vi "Generate Process.vi"(8 "error in (no error)":errorcluster, 11 "Process Generator In":refnum<class "Process Generator.lvclass">) -> (0 "error out":errorcluster, 3 "Process Generator Out":refnum<class "Process Generator.lvclass">)   [LabVIEW 2020, in "Process Generator.lvclass"]
uses:
  Process Generator.lvclass
  Process Generator.lvclass/Process Generator.ctl
  Framework/Process/Process.lvclass
  C:/Users/anton/Documents/GitHub/Triarc-Framework/source/Framework/Base/Base.lvclass
  C:/Users/anton/Documents/GitHub/Triarc-Framework/source/Framework/Configuration File/Configuration File.lvclass
  C:/Users/anton/Documents/GitHub/Triarc-Framework/source/Framework/Process/Process.lvclass
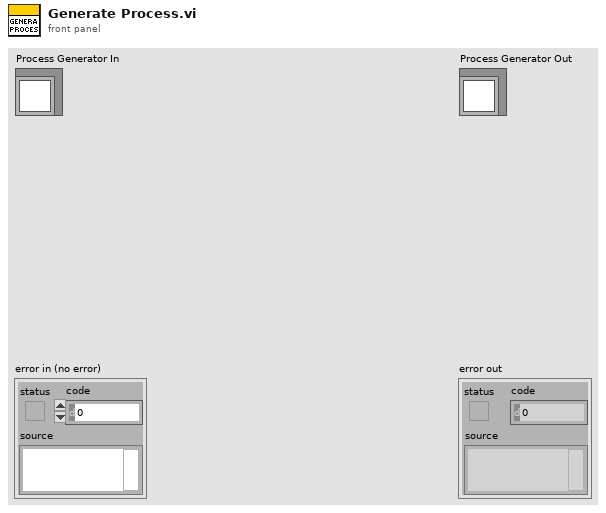
[diagram p1: front panel]
types:
  T1 = enum32{"invalid scope", "public", "private", "protected", "community"}[]
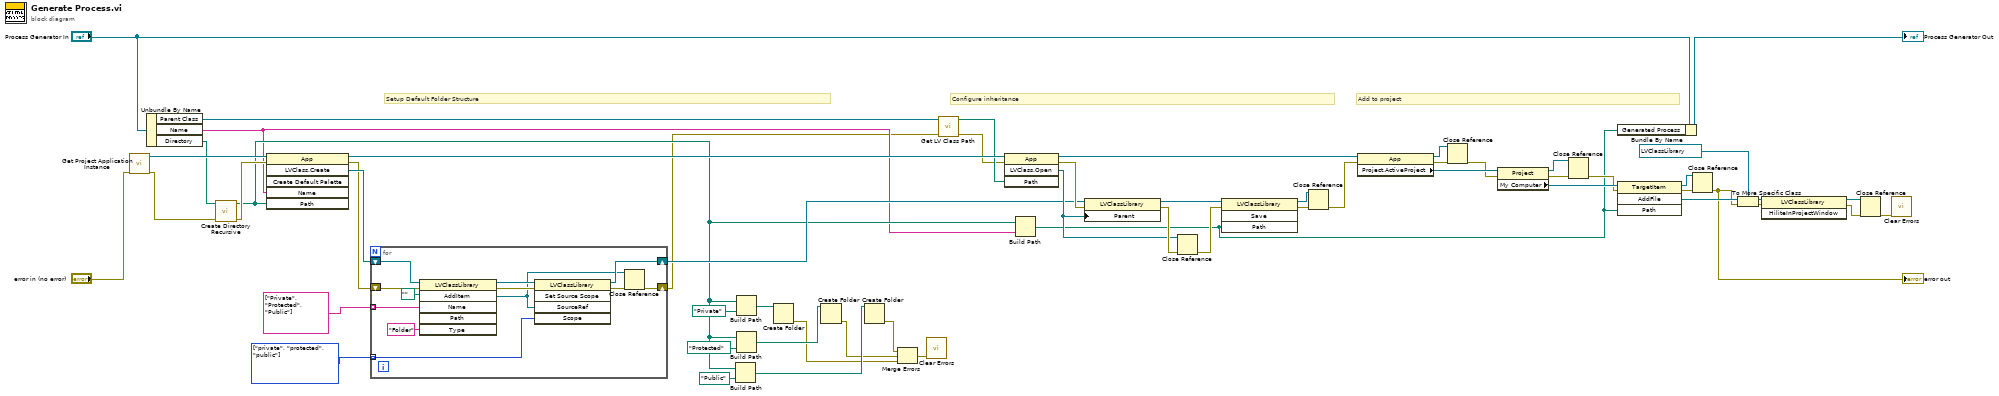
[diagram p0: block diagram]
diagram:
  w28 = T1 [enum."private", enum."protected", enum."public"] items=["invalid scope", "public", "private", "protected", "community"] ("scope")
  # "Add to project"
  # "Configure inheritance"
  # "Setup Default Folder Structure"
  n1 = call "Get Project Application Instance.vi"("error in (no error)"="error in (no error)") -> ("error out"=w20:errorcluster, "Application out"=w22:refnum<vi>)  [unwired: 9 in]
  n2 = Unbundle By Name("Process Generator In") -> ("Parent Class"=w56:refnum<class "Process.lvclass">, "Name"=w15:string, "Directory"=w14:path)
  n3 = call <vilib>:"Create Directory Recursive.vi"("error in (no error)"=w20, "directory"=w14) -> ("error out"=w41:errorcluster, "directory copy"=w17:path)  [unwired: 3 in, 1 out]
  n4 = invoke class="App" method="LVClass.Create"(reference=w22, error in=w41, "Name"=w15, "Path"=w17) -> (reference out=w55:refnum<vi>, error out=w26:errorcluster, "LVClass.Create"=w29:refnum<vi>)  [unwired: 2 in, 3 out]
  n5 = for {
    tunnel: string[] ["Private", "Protected", "Public"] ("Name") -> [w69] mode=indexing
    tunnel: w28 -> [w64] mode=indexing
    shift-right: [w63] -> w27
    shift-left: w29 -> [w67]
    shift-right: [w59] -> w13
    shift-left: w26 -> [w61]
    n6 = invoke class="LVClassLibrary" method="AddItem"(reference=w67, error in=w61, "Name"=w69, "Path"=path "", "Type"="Folder") -> (reference out=w65:refnum<vi>, error out=w62:errorcluster, "AddItem"=w58:refnum<vi>)  [unwired: 1 in, 3 out]
    n7 = invoke class="LVClassLibrary" method="Set Source Scope"(reference=w65, error in=w62, "SourceRef"=w58, "Scope"=w64) -> (reference out=w63:refnum<vi>, error out=w60:errorcluster)  [unwired: 1 in, 3 out]
    n8 = Close Reference(reference=w58, error in (no error)=w60) -> (error out=w59:errorcluster)
  }
  n9 = Build Path(base path=w17, name or relative path=path "Public") -> (appended path=w16:path)
  n10 = Build Path(base path=w17, name or relative path=path "Private") -> (appended path=w24:path)
  n11 = Build Path(base path=w17, name or relative path=path "Protected") -> (appended path=w23:path)
  n12 = Create Folder(path (use dialog)=w24) -> (error out=w10:errorcluster)  [unwired: 2 in, 2 out]
  n13 = Create Folder(path (use dialog)=w23) -> (error out=w11:errorcluster)  [unwired: 2 in, 2 out]
  n14 = Create Folder(path (use dialog)=w16) -> (error out=w12:errorcluster)  [unwired: 2 in, 2 out]
  n15 = Merge Errors(w12, w11, w10) -> (w9:errorcluster)
  n16 = call <vilib>:"Clear Errors.vi"("error in (no error)"=w9) -> ()  [unwired: 5 in, 2 out]
  n17 = call <vilib>:"Get LV Class Path.vi"("error in (no error)"=w13, "object"=w56) -> ("error out"=w40:errorcluster, "class path"=w54:path)  [unwired: 8 in]
  n18 = invoke class="App" method="LVClass.Open"(reference=w55, error in=w40, "Path"=w54) -> (reference out=w52:refnum<vi>, error out=w53:errorcluster, "LVClass.Open"=w33:refnum<vi>)  [unwired: 1 in, 1 out]
  n19 = Build Path(base path=w17, name or relative path=w15) -> (appended path=w31:path)
  n20 = property class="LVClassLibrary"(reference=w27, error in=w53, "Parent"=w33) -> (reference out=w48:refnum<vi>, error out=w47:errorcluster)
  n21 = Close Reference(reference=w33, error in (no error)=w47) -> (error out=w34:errorcluster)
  n22 = invoke class="LVClassLibrary" method="Save"(reference=w48, error in=w34, "Path"=w31) -> (reference out=w44:refnum<vi>, error out=w46:errorcluster)  [unwired: 1 in, 2 out]
  n23 = Close Reference(reference=w44, error in (no error)=w46) -> (error out=w45:errorcluster)
  n24 = property class="App"(reference=w52, error in=w45) -> (reference out=w38:refnum<vi>, error out=w50:errorcluster, "Project.ActiveProject"=w51:refnum<vi>)
  n25 = Close Reference(reference=w38, error in (no error)=w50) -> (error out=w39:errorcluster)
  n26 = property class="Project"(reference=w51, error in=w39) -> (reference out=w36:refnum<vi>, error out=w43:errorcluster, "My Computer"=w49:refnum<vi>)
  n27 = Close Reference(reference=w36, error in (no error)=w43) -> (error out=w37:errorcluster)
  n28 = invoke class="TargetItem" method="AddFile"(reference=w49, error in=w37, "Path"=w31) -> (reference out=w35:refnum<vi>, error out=w42:errorcluster, "AddFile"=w6:refnum<vi>)  [unwired: 1 in, 1 out]
  n29 = Bundle By Name(cluster="Process Generator In", "Generated Process"=w31) -> (→"Process Generator Out":refnum<class "Process Generator.lvclass">)
  n30 = Close Reference(reference=w35, error in (no error)=w42) -> (error out=w5:errorcluster)
  "error out" <- w5
  n31 = To More Specific Class(target class=refnum<vi> refnum ("reference"), reference=w6, error in=w5) -> (specific class reference=w8:refnum<vi>, error out=w4:errorcluster)
  n32 = invoke class="LVClassLibrary" method="HiliteInProjectWindow"(reference=w8, error in=w4) -> (reference out=w2:refnum<vi>, error out=w3:errorcluster)  [unwired: 1 in, 1 out]
  n33 = Close Reference(reference=w2, error in (no error)=w3) -> (error out=w1:errorcluster)
  n34 = call <vilib>:"Clear Errors.vi"("error in (no error)"=w1) -> ()  [unwired: 5 in, 2 out]
